vi "PV MiniTest Measure.vi"(8 "error in (no error)":errorcluster, 9 "MiniTest Measure - Cluster":T1={"Parameter"=5, "Parameter\nread only<->describe"=FALSE, "Value in"=1e-09} {"Value in" min=1e-09 max=100000.0 step=1e-09 format="%.2e"; "Parameter" items=[" Pressure of the ext. Gauge [mbar] (read only)", " Zero (update background suppression)", " Leakrate [selected unit] (read only)", " Leakrate  [mbarl/s] (read only)", " Leakrate of external test leak [selected unit] (read only)", " Pressure internal sensor [selected unit] (read only)", " Trigger [selected unit]", " Trigger [mbar l/s]", " Pressure of the ext. Gauge [selected unit] (read only]", " Gauge Type (read only)"]}, 10 "Adress of unit":u16=1 min=1 max=999 step=1, 11 "VISA session":refnum<visa-resource-name>) -> (0 "error out":errorcluster, 2 "response (data)":string, 3 "dup VISA session":refnum<visa-resource-name>)   [LabVIEW 2016, in "Pfeiffer Vacuum.lvlib"]
doc: "There are 10 parameters available, only one of which can be enabled at a time. \n\n0 - Pressure of the ext. Gauge [mbar] (read only) - Para 340\n1 - Zero (update background suppression) - Para 651\n2 - Leakrate [selected unit] (read only) - Para 669\n3 - Leakrate [mbarl/s] (read only) - Para 670\n4 - Leakrate of external test leak [selected unit] (read only) - Para 671\n5 - Pressure internal sensor [selected unit] (read only) - Para 679\n6 - Trigger [selected unit] - Para 681\n7 - Trigger [mbar l/s] - Para 682\n8 - Pressure of the ext. Gauge [selected unit] (read only] - Para 690\n9 - Gauge Type (read only) - Para 738\n\nNote: The one control right of this one will set the appropriate values for the selected parameter. Any settings for an parameter that is not selected will be ignored. If a value is out of range, it will be changed to either the upper or the lower limit of the range."
uses:
  Pfeiffer Vacuum.lvlib
  PV MiniTest Measure - Cluster.ctl
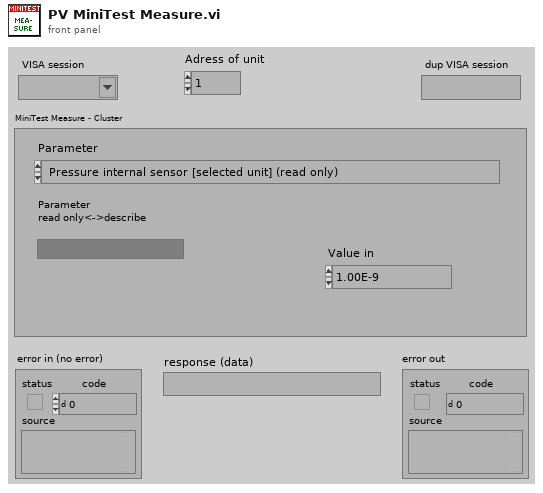
[diagram p1: front panel]
types:
  T1 = typedef "Pfeiffer Vacuum.lvlib/PV MiniTest Measure - Cluster.ctl" = cluster{"Parameter":u16, "Parameter\nread only<->describe":bool, "Value in":dbl}
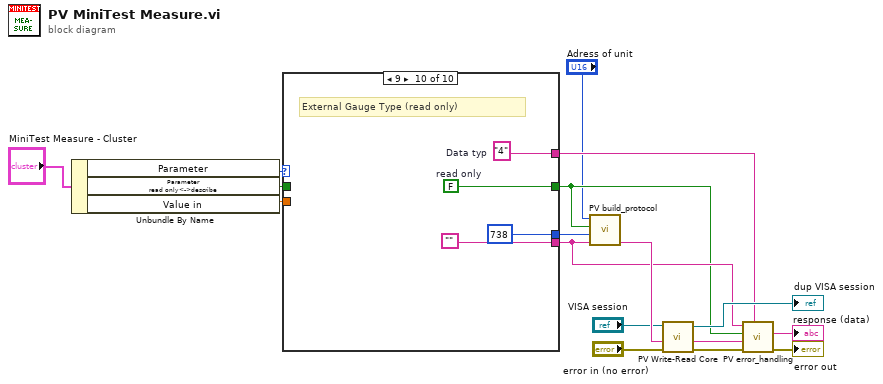
[diagram p0: block diagram]
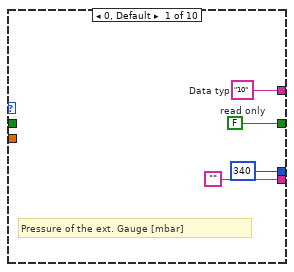
[diagram p2: hidden frame]
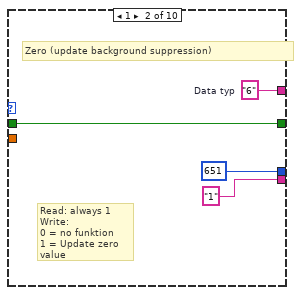
[diagram p3: hidden frame]
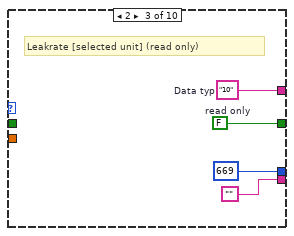
[diagram p4: hidden frame]
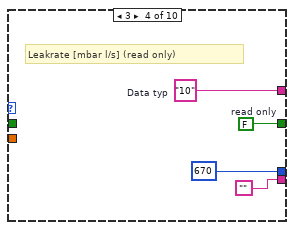
[diagram p5: hidden frame]
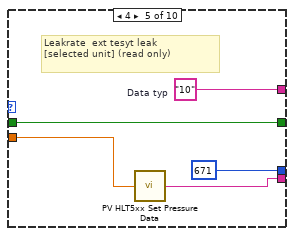
[diagram p6: hidden frame]
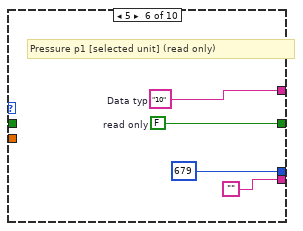
[diagram p7: hidden frame]
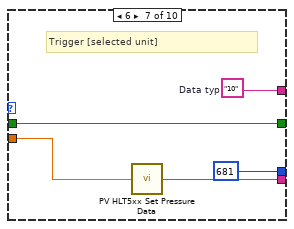
[diagram p8: hidden frame]
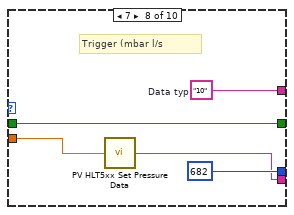
[diagram p9: hidden frame]
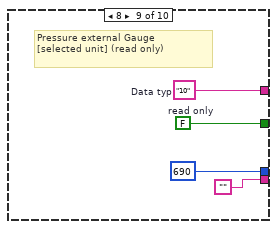
[diagram p10: hidden frame]
diagram:
  n1 = Unbundle By Name("MiniTest Measure - Cluster") -> ("Parameter"=w5:u16, "Parameter\nread only<->describe"=w16:bool, "Value in"=w1:dbl)
  n2 = case shown="9" w5 {
    tunnel: [u16 340 ("Parameter-number") u16 651 ("Parameter-number") u16 669 ("Parameter-number") u16 670 ("Parameter-number") u16 671 ("Parameter-number") u16 679 ("Parameter-number") u16 681 ("Parameter-number") u16 682 ("Parameter-number") u16 690 ("Parameter-number") u16 738 ("Parameter-number")] -> w17
    tunnel: ["" "1" ("Data") "" "" w34 "" w44 w49 "" ""] -> w12
    tunnel: [w19 w23 w28 w30 w36 w41 w45 w48 w54 w57] -> w10
    tunnel: w16 -> [_ w23 _ _ w36 _ w45 w48 _ _]
    tunnel: [w21 w22 w29 w33 w38 w42 w47 w52 w56 w60] -> w11
    tunnel: w1 -> [_ _ _ _ w35 _ w43 w50 _ _]
    frame 0, Default {
      w19 = FALSE  # read only
      w21 = "10"  # Data typ
      # "Pressure of the ext. Gauge [mbar]"
    }
    frame 1 {
      w22 = "6"  # Data typ
      # "Read: always 1\nWrite:\n0 = no funktion\n1 = Update zero value"
      # "Zero (update background suppression)"
    }
    frame 2 {
      w29 = "10"  # Data typ
      w28 = FALSE  # read only
      # "Leakrate [selected unit] (read only)"
    }
    frame 3 {
      w30 = FALSE  # read only
      w33 = "10"  # Data typ
      # "Leakrate [mbar l/s] (read only)"
    }
    frame 4 {
      w38 = "10"  # Data typ
      # "Leakrate  ext tesyt leak\n[selected unit] (read only)"
      n3 = call "PV HLT5xx Set Pressure Data.vi"("Value in"=w35) -> ("Output"=w34:string)
    }
    frame 5 {
      w42 = "10"  # Data typ
      w41 = FALSE  # read only
      # "Pressure p1 [selected unit] (read only)"
    }
    frame 6 {
      w47 = "10"  # Data typ
      # "Trigger [selected unit]"
      n4 = call "PV HLT5xx Set Pressure Data.vi"("Value in"=w43) -> ("Output"=w44:string)
    }
    frame 7 {
      w52 = "10"  # Data typ
      # "Trigger (mbar l/s"
      n5 = call "PV HLT5xx Set Pressure Data.vi"("Value in"=w50) -> ("Output"=w49:string)
    }
    frame 8 {
      w54 = FALSE  # read only
      w56 = "10"  # Data typ
      # "Pressure external Gauge\n[selected unit] (read only)"
    }
    frame 9 {
      w57 = FALSE  # read only
      w60 = "4"  # Data typ
      # "External Gauge Type (read only)"
    }
  }
  n6 = call "PV build_protocol.vi"("Data"=w12, "Parameter-number"=w17, "parameter\nread<->describe"=w10, "Adress"="Adress of unit") -> ("output"=w15:string)  [unwired: 3 in]
  n7 = call "PV Write-Read Core.vi"("error in"="error in (no error)", "Write data in"=w15, "VISA session"="VISA session") -> ("error out"=w14:errorcluster, "response (data) out"=w3:string, "dup VISA session"=→"dup VISA session":refnum<visa-resource-name>)  [unwired: 2 in]
  n8 = call "PV error_handling.vi"("Data Typ in"=w11, "error in"=w14, "response (data) in"=w3, "Parameter\nread only<->describe"=w10, "data in"=w12) -> ("error out"=→"error out":errorcluster, "Data out"=→"response (data)":string)  [unwired: 4 in, 1 out]
